vi "Get Collatz sequence-without array output.vi"(8 "error in (no error)":errorcluster, 11 "n = starting term":i32) -> (0 "error out":errorcluster, 2 "no. of elements (chain length)":i32)   [LabVIEW 2021, in "Numeric Utilities.lvlib"]
uses:
  Numeric Utilities.lvlib
panel:
  in  "Dev: stop early":bool
  out "iteration":i32
  # "Development\ncontrols/indicators useful for development and testing, but which are not outputs of the VI"
  # "Input\nInputs to the VI"
  # "Output\nOutputs of the VI"
  # "Description"
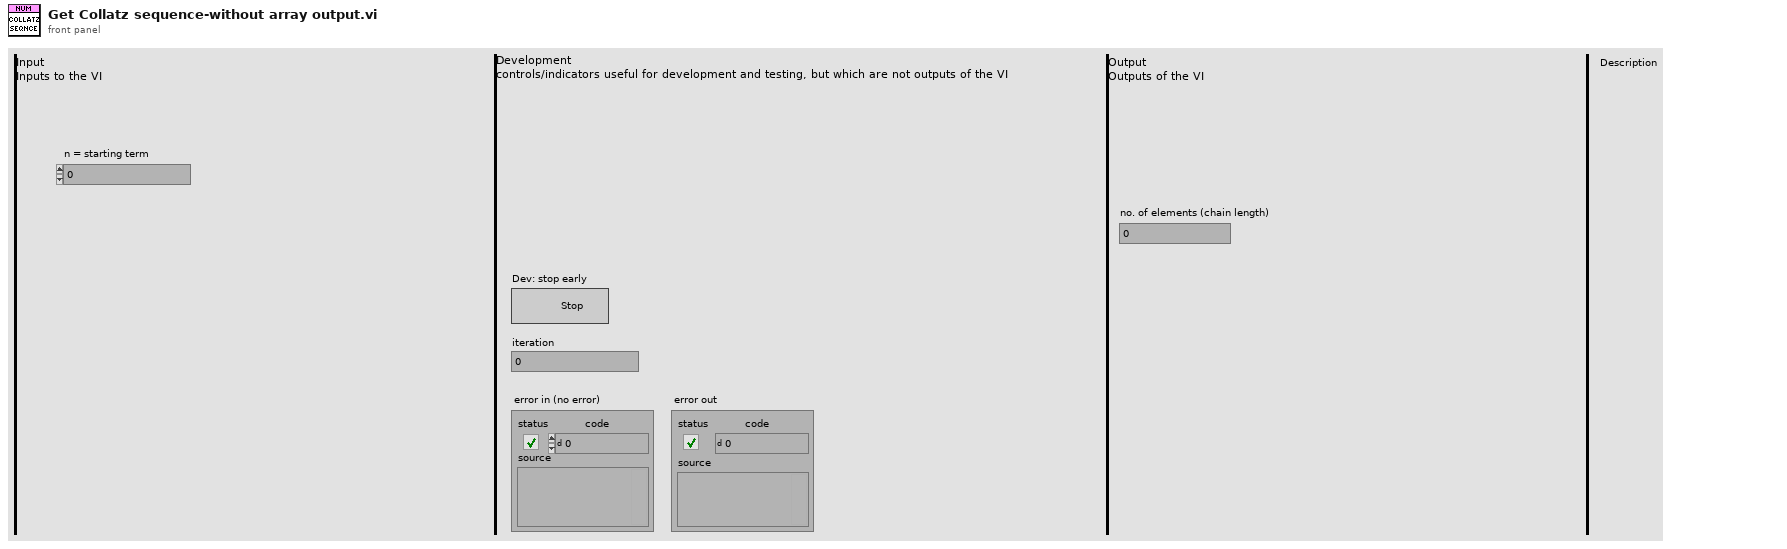
[diagram p1: front panel]
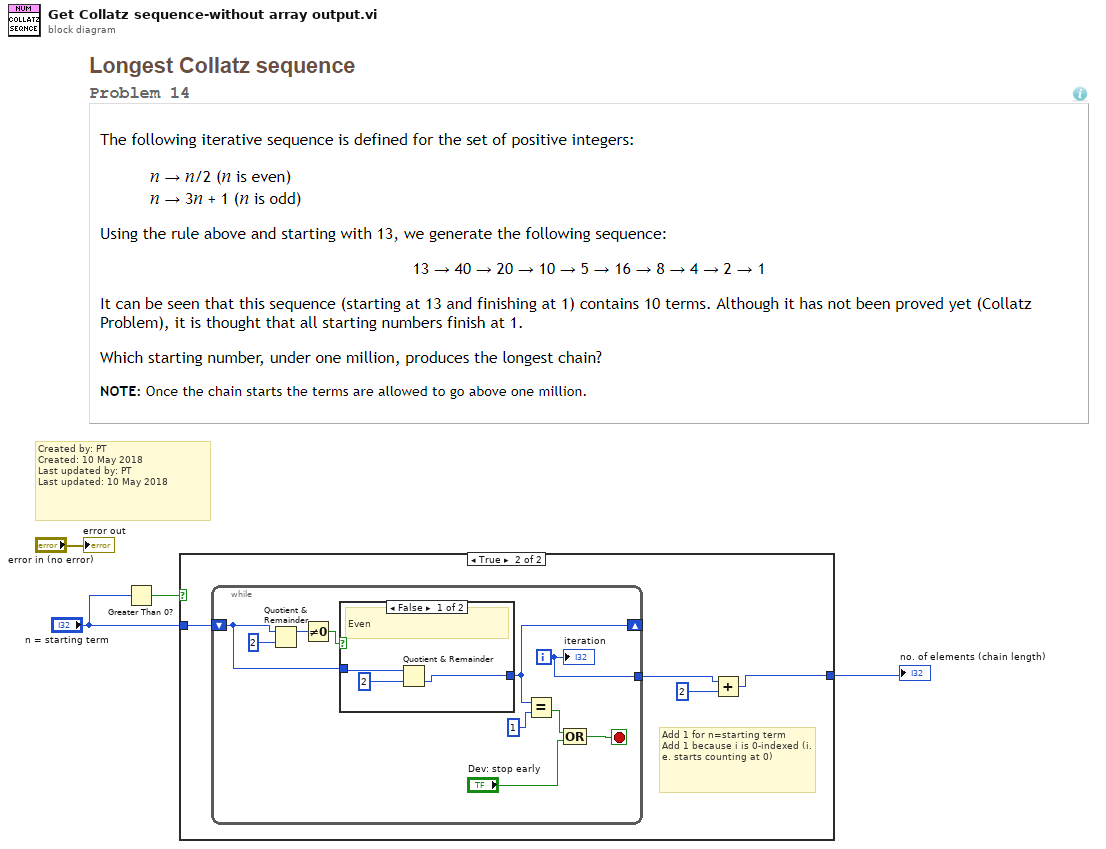
[diagram p0: block diagram]
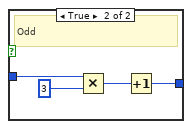
[diagram p3: hidden frame]
diagram:
  # "Created by: PT\nCreated: 10 May 2018\nLast updated by: PT\nLast updated: 10 May 2018"
  n1 = Greater Than 0?(x="n = starting term") -> (x > 0?=w3:bool)
  n2 = case shown="True" w3 {
    tunnel: "n = starting term" -> [_ w8]
    tunnel: [_ w5] -> w1
    frame False {
    }
    frame True {
      # "Add 1 for n=starting term\nAdd 1 because i is 0-indexed (i.e. starts counting at 0)"
      n3 = while {
        shift-right: [w17] -> _
        shift-left: w8 -> [w9]
        tunnel: [w13] -> w7
        i -> [w13]
        stop <- w15 stop-if-true
        n4 = Quotient & Remainder(x=w9, y=2) -> (x-y*floor(x/y)=w12:i32)  [unwired: 1 out]
        n5 = Not Equal To 0?(x=w12) -> (x != 0?=w10:bool)
        n6 = case shown="False" w10 {
          tunnel: w9 -> [w21 w25]
          tunnel: [w19 w22] -> w17
          frame False {
            # "Even"
            n7 = Quotient & Remainder(x=w21, y=2) -> (floor(x/y)=w19:i32)  [unwired: 1 out]
          }
          frame True {
            # "Odd"
            n8 = Multiply(x=w25, y=3) -> (x*y=w23:i32)
            n9 = Increment(x=w23) -> (x+1=w22:i32)
          }
        }
        n10 = Equal?(x=w17, y=1) -> (x = y?=w16:bool)
        n11 = Compound Arithmetic op=OR(w16, "Dev: stop early") -> (w15:bool)
        "iteration" <- w13
      }
      n12 = Add(x=w7, y=2) -> (x+y=w5:i32)
    }
  }
  "no. of elements (chain length)" <- w1
  "error out" <- "error in (no error)"
